vi "IMIC_GetXYPos.vi"(0 "handle":u64) -> (1 "output param":T1(ring), 2 "handle out":u64, 3 "xpos":dbl, 4 "ypos":dbl)   [LabVIEW 2011]
uses:
  tillimic32.dll
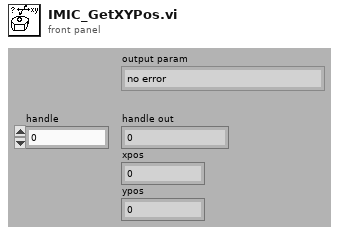
[diagram p1: front panel]
types:
  T1 = enum16{"no error", "missing axis", "missing Z axis", "missing Filter", "iMic not initialized", "no property", "wrong handle", "protocol not finished", "user parameter to long (>32 bits)", "no user parameter handle", "failed to open comport", "failed to initialize"}
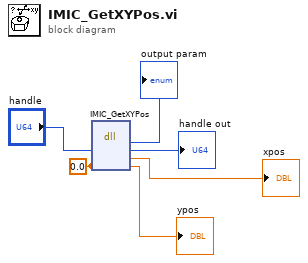
[diagram p0: block diagram]
diagram:
  w1 = 0.0 ("zpos")
  n1 = dll-call lib="D:/Colibri/Drivers/TILLPhotonics/tillimic*.*" fn="IMIC_GetXYPos"("handle"="handle", "xpos"=w1, "ypos"=w1) -> ("return type"=→"output param":i32, "handle"=→"handle out":u64, "xpos"=→"xpos":dbl, "ypos"=→"ypos":dbl)  [unwired: 3 in, 2 out]
